vi "EXETest.vi"() -> ()   [LabVIEW 2013]
panel:
  in  "End Program":bool
  out "Boolean 2":bool
  in  "Boolean":bool
  out "Numeric 2":dbl
  in  "Numeric":dbl
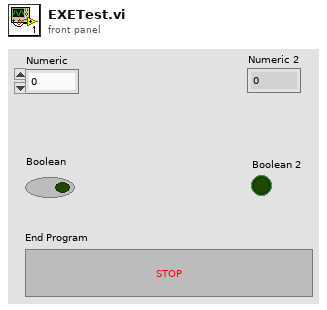
[diagram p1: front panel]
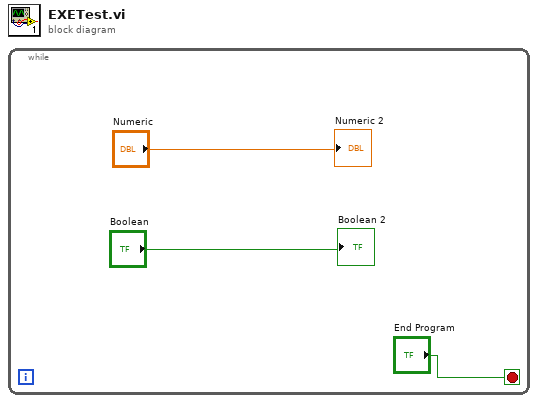
[diagram p0: block diagram]
diagram:
  n1 = while {
    stop <- "End Program" stop-if-true
    "Numeric 2" <- "Numeric"
    "Boolean 2" <- "Boolean"
  }
